vi "Database.Init.vi"(8 "error in (no error)":errorcluster) -> (0 "error out":errorcluster)   [LabVIEW 2016]
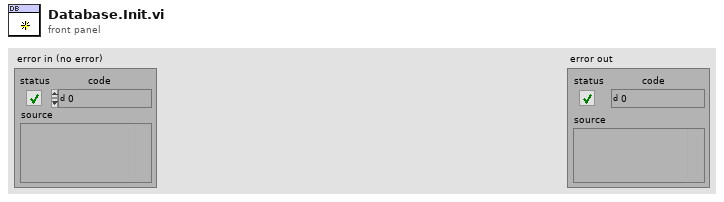
[diagram p1: front panel]
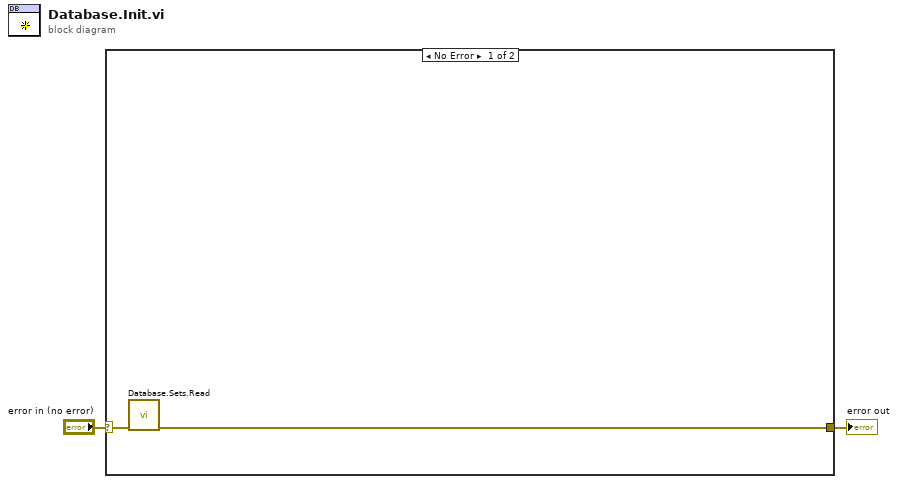
[diagram p0: block diagram]
diagram:
  n1 = case shown="No Error" "error in (no error)" {
    selector: "error in (no error)" -> [w4 w5]
    tunnel: [w3 w5] -> w1
    frame No Error {
      n2 = call "Database.Sets.Read.vi"("error in"=w4) -> ("error out"=w3:errorcluster)  [unwired: 10 in]
    }
    frame Error {
    }
  }
  "error out" <- w1
